vi "ESP32_initialize.vi"(0 "ESP32 IN":refnum<visa-resource-name>, 1 "Switch On Time":u8 caption="Switch On Time(uS)", 2 "Switch Off Time":u8=100 caption="Switch Off Time(uS)", 3 "Enable Accurate \nMeasure":bool=TRUE, 11 "error in (no error)":errorcluster, 12 "Measure Current \nOnly":bool=TRUE, 13 "Scan Measure\nTime(uS)":i32=100, 14 "Sample number":i32=1) -> (4 "ESP32 out":refnum<visa-resource-name>, 15 "error out":errorcluster)   [LabVIEW 2023]
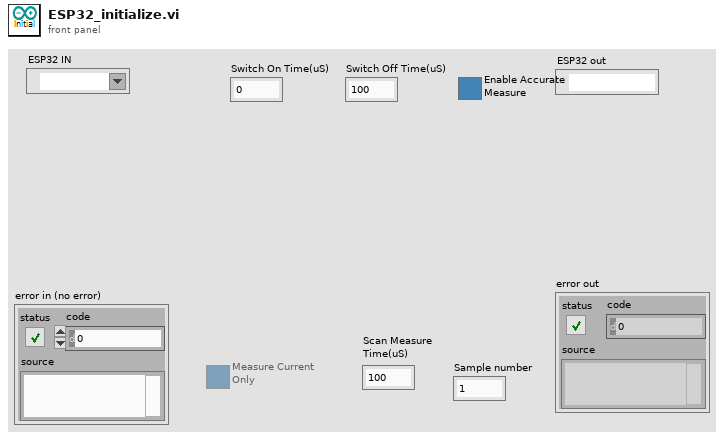
[diagram p1: front panel]
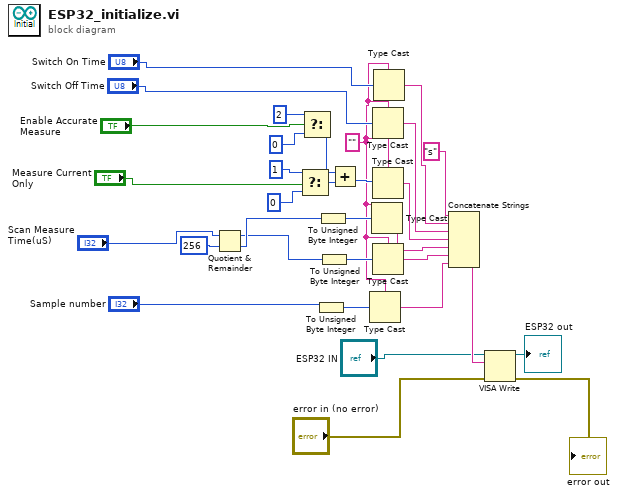
[diagram p0: block diagram]
diagram:
  w3 = "" ("string")
  n1 = Quotient & Remainder(x="Scan Measure\nTime(uS)", y=u32 256) -> (x-y*floor(x/y)=w9:u32, floor(x/y)=w23:u32)
  n2 = Select(t=u8 1, s="Measure Current \nOnly", f=u8 0) -> (s? t:f=w20:u8)
  n3 = Select(t=u8 2, s="Enable Accurate \nMeasure", f=u8 0) -> (s? t:f=w21:u8)
  n4 = To Unsigned Byte Integer(number="Sample number") -> (unsigned 8bit integer=w4:u8)
  n5 = To Unsigned Byte Integer(number=w23) -> (unsigned 8bit integer=w27:u8)
  n6 = To Unsigned Byte Integer(number=w9) -> (unsigned 8bit integer=w31:u8)
  n7 = Add(x=w21, y=w20) -> (x+y=w19:u8)
  n8 = Type Cast(type=w3, x=w4) -> (*(type *) &x=w1:string)
  n9 = Type Cast(type=w3, x=w27) -> (*(type *) &x=w28:string)
  n10 = Type Cast(type=w3, x="Switch Off Time") -> (*(type *) &x=w15:string)
  n11 = Type Cast(type=w3, x=w19) -> (*(type *) &x=w29:string)
  n12 = Type Cast(type=w3, x=w31) -> (*(type *) &x=w32:string)
  n13 = Type Cast(type=w3, x="Switch On Time") -> (*(type *) &x=w16:string)
  n14 = Concatenate Strings("s" ("data in"), w16, w15, w29, w28, w32, w1) -> (w30:string)
  n15 = VISA Write(VISA resource name="ESP32 IN", write buffer=w30, error in (no error)="error in (no error)") -> (VISA resource name out=→"ESP32 out":refnum<visa-resource-name>, error out=→"error out":errorcluster)  [unwired: 1 out]
